vi "State Machine - Enqueue State.vi"(6 "Front?":bool, 8 "error in (no error)":errorcluster, 9 "Data":variant, 10 "State":string, 11 "Queue In":refnum<queue>) -> (0 "error out":errorcluster, 3 "Queue Out":refnum<queue>)   [LabVIEW 2015, in "State Machine.lvlib"]
uses:
  State Machine.lvlib
  Controls/Message.ctl
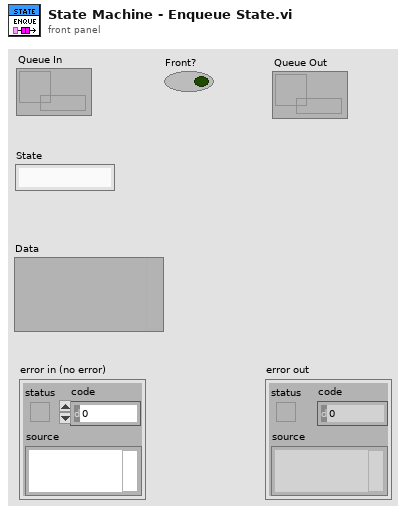
[diagram p1: front panel]
types:
  T1 = typedef "State Machine.lvlib/Message.ctl" = cluster{"State":string, "Data":variant}
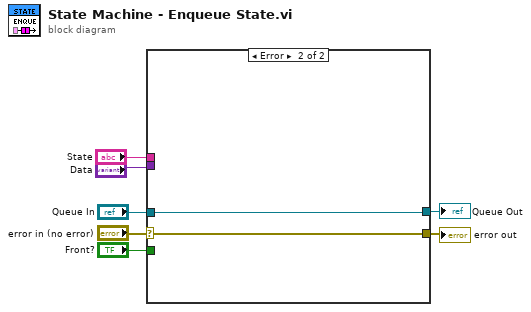
[diagram p0: block diagram]
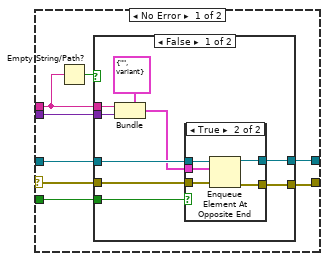
[diagram p2: hidden frame]
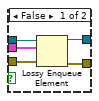
[diagram p3: hidden frame]
diagram:
  n1 = case shown="Error" "error in (no error)" {
    selector: "error in (no error)" -> [w15 w38]
    tunnel: [w11 w38] -> w7
    tunnel: "State" -> [w9 _]
    tunnel: "Data" -> [w14 _]
    tunnel: "Queue In" -> [w13 w37]
    tunnel: "Front?" -> [w12 _]
    tunnel: [w8 w37] -> w1
    frame No Error {
      n2 = Empty String/Path?(string/path=w9) -> (empty?=w10:bool)
      n3 = case shown="False" w10 {
        tunnel: w15 -> [w24 w36]
        tunnel: w9 -> [w22 _]
        tunnel: w14 -> [w21 _]
        tunnel: w13 -> [w20 w35]
        tunnel: w12 -> [w18 _]
        tunnel: [w17 w36] -> w11
        tunnel: [w16 w35] -> w8
        frame False {
          n4 = Bundle(cluster=T1 {"State"="", "Data"=variant} ("Message"), "State"=w22, "Data"=w21) -> (w19:T1)
          n5 = case shown="True" w18 {
            tunnel: w24 -> [w29 w31]
            tunnel: w20 -> [w28 w34]
            tunnel: w19 -> [w27 w32]
            tunnel: [w26 w33] -> w16
            tunnel: [w25 w30] -> w17
            frame False {
              n6 = Lossy Enqueue Element(queue=w28, element=w27, error in (no error)=w29) -> (queue out=w26:refnum<queue>, error out=w25:errorcluster)  [unwired: 2 out]
            }
            frame True {
              n7 = Enqueue Element At Opposite End(queue=w34, element=w32, error in (no error)=w31) -> (queue out=w33:refnum<queue>, error out=w30:errorcluster)  [unwired: 1 in, 1 out]
            }
          }
        }
        frame True {
        }
      }
    }
    frame Error {
    }
  }
  "error out" <- w7
  "Queue Out" <- w1
